vi "q2 file read case conversion.vi"() -> ()   [LabVIEW 2025]
panel:
  out "all upper case string":string
  out "text":string
  in  "output path":path
  in  "input path":path
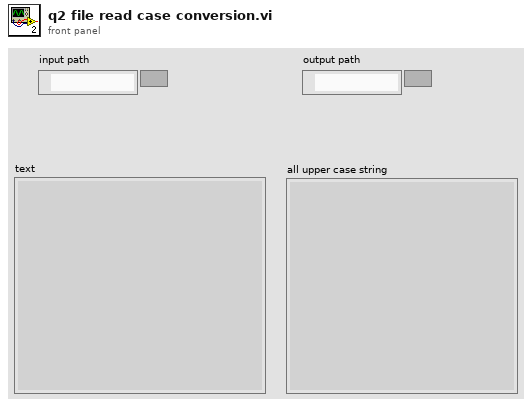
[diagram p1: front panel]
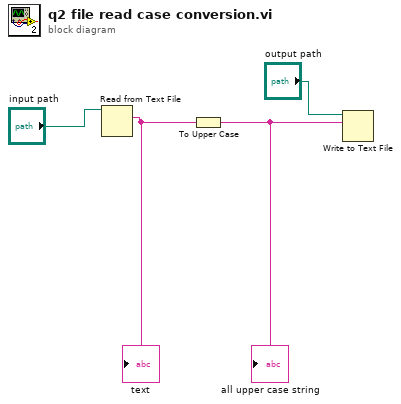
[diagram p0: block diagram]
diagram:
  n1 = Read from Text File(file (use dialog)="input path") -> (text=w3:string)  [unwired: 3 in, 3 out]
  "text" <- w3
  n2 = To Upper Case(1:w3) -> (0:w2:string)
  "all upper case string" <- w2
  n3 = Write to Text File(file (use dialog)="output path", text=w2) -> ()  [unwired: 2 in, 3 out]
